vi "Complex to DB.vi"(8 "error in (no error)":errorcluster, 11 "Complix FFT In":refnum<class "2D Array c32.lvclass">) -> (0 "error out":errorcluster, 3 "Db Amplitude Out":refnum<class "2D Array f32.lvclass">)   [LabVIEW 2020, in "Signal Analysis.lvlib" / "Signal Analysis.lvclass"]
uses:
  Signal Analysis.lvclass
  <vilib>/Natan Biesmans/G2CPU GPU and CPU HPC Toolkit/G2CPU Libraries/Arrays/2DArray/c32/2D Array c32.lvclass
  C:/Program Files/National Instruments/LabVIEW 2025/vi.lib/Natan Biesmans/G2CPU GPU and CPU HPC Toolkit/G2CPU Libraries/Arrays/Array/Array Prototype.lvclass
  <vilib>/Natan Biesmans/G2CPU GPU and CPU HPC Toolkit/G2CPU Libraries/Arrays/2DArray/f32/2D Array f32.lvclass
  ae8c32fd-c519-49ae-a133-193997b97273.vi
  5b3a9c71-2296-4b0e-aa5a-23b530eb68bb.vi
  9631c890-40d0-4dd2-8f0c-9650434c6622.vi
  71c5292d-49ae-4f2f-bdc5-1c901a887993.vi
  ae8c32fd-c519-49ae-a133-193997b97273.vi/b6535cc3-4f5d-45ad-9052-c08cd62b0315.vi
  ae8c32fd-c519-49ae-a133-193997b97273.vi/c9d07b13-7729-4cda-a81e-7ca6043257da.vi
  ae8c32fd-c519-49ae-a133-193997b97273.vi/4470c8c9-d353-49e9-bc1e-f4fe0b2204ee.vi
  ae8c32fd-c519-49ae-a133-193997b97273.vi/b48f0110-6046-499d-b6aa-1db73cdea65c.vi
  5b3a9c71-2296-4b0e-aa5a-23b530eb68bb.vi/def40612-844c-421c-bb75-87c330777b0b.vi
  9631c890-40d0-4dd2-8f0c-9650434c6622.vi/31b317ac-79b4-42cb-9c55-b9b94a2bc574.vi
  71c5292d-49ae-4f2f-bdc5-1c901a887993.vi/6197f869-f6d4-49b3-9b2c-cc979b422c2e.vi
  71c5292d-49ae-4f2f-bdc5-1c901a887993.vi/a7e86dbb-b4c0-485c-89c5-522e60ee265c.vi
  71c5292d-49ae-4f2f-bdc5-1c901a887993.vi/6197f869-f6d4-49b3-9b2c-cc979b422c2e.vi/2c12aba4-aacf-4d7a-adbe-039f6155a93e.vi
  71c5292d-49ae-4f2f-bdc5-1c901a887993.vi/6197f869-f6d4-49b3-9b2c-cc979b422c2e.vi/f38cccb2-46f6-49f0-a8d6-9da0c88ff6f3.vi
  71c5292d-49ae-4f2f-bdc5-1c901a887993.vi/6197f869-f6d4-49b3-9b2c-cc979b422c2e.vi/bdde7ba0-fc5a-4512-a8ec-1695e5fcee25.vi
  71c5292d-49ae-4f2f-bdc5-1c901a887993.vi/6197f869-f6d4-49b3-9b2c-cc979b422c2e.vi/3e802c67-fb96-46a3-ae13-4994a8508b4f.vi
  71c5292d-49ae-4f2f-bdc5-1c901a887993.vi/6197f869-f6d4-49b3-9b2c-cc979b422c2e.vi/5a50fc67-79e7-4972-80c2-92243cd53dd4.vi
  71c5292d-49ae-4f2f-bdc5-1c901a887993.vi/a7e86dbb-b4c0-485c-89c5-522e60ee265c.vi/730f6c57-5c0b-4ee9-b61e-75067b25222b.vi
  71c5292d-49ae-4f2f-bdc5-1c901a887993.vi/a7e86dbb-b4c0-485c-89c5-522e60ee265c.vi/096b8799-7810-404e-baca-ba9279cec4bd.vi
  71c5292d-49ae-4f2f-bdc5-1c901a887993.vi/a7e86dbb-b4c0-485c-89c5-522e60ee265c.vi/0f1a5a47-bcc5-4796-ac31-8dfcfbc0d7d1.vi
  71c5292d-49ae-4f2f-bdc5-1c901a887993.vi/a7e86dbb-b4c0-485c-89c5-522e60ee265c.vi/89f12e17-3330-4b72-ad8f-8dd636660732.vi
  71c5292d-49ae-4f2f-bdc5-1c901a887993.vi/6197f869-f6d4-49b3-9b2c-cc979b422c2e.vi/5a50fc67-79e7-4972-80c2-92243cd53dd4.vi/1b7cf390-2ae0-48f3-9bce-03c57eed6ee8.vi
  <vilib>/Natan Biesmans/G2CPU GPU and CPU HPC Toolkit/G2CPU Libraries/Arrays/1DArray/f32/1D Array f32.lvclass
  <vilib>/Natan Biesmans/G2CPU GPU and CPU HPC Toolkit/G2CPU Libraries/Arrays/Array/G2CPU Lock Array.vi
  <vilib>/Natan Biesmans/G2CPU GPU and CPU HPC Toolkit/G2CPU Libraries/Arrays/Array/G2CPU Get Array Pointer.vi
  <vilib>/Natan Biesmans/G2CPU GPU and CPU HPC Toolkit/ArrayFire Driver/VIs/real.vi
  <vilib>/Natan Biesmans/G2CPU GPU and CPU HPC Toolkit/ArrayFire Driver/VIs/imag.vi
  <vilib>/Natan Biesmans/G2CPU GPU and CPU HPC Toolkit/ArrayFire Driver/VIs/hypot.vi
  <vilib>/Natan Biesmans/G2CPU GPU and CPU HPC Toolkit/ArrayFire Driver/VIs/release array.vi
  <vilib>/Natan Biesmans/G2CPU GPU and CPU HPC Toolkit/ArrayFire Driver/VIs/arg.vi
  <vilib>/Natan Biesmans/G2CPU GPU and CPU HPC Toolkit/G2CPU Libraries/Arrays/Array/G2CPU Set Array Pointer.vi
  <vilib>/Natan Biesmans/G2CPU GPU and CPU HPC Toolkit/G2CPU Libraries/Arrays/Array/G2CPU Unlock Array.vi
  <vilib>/Natan Biesmans/G2CPU GPU and CPU HPC Toolkit/ArrayFire Driver/VIs/abs.vi
  <vilib>/Natan Biesmans/G2CPU GPU and CPU HPC Toolkit/ArrayFire Driver/VIs/log10.vi
  <vilib>/Natan Biesmans/G2CPU GPU and CPU HPC Toolkit/ArrayFire Driver/VIs/Run as Multi Device.vi
  <vilib>/Natan Biesmans/G2CPU GPU and CPU HPC Toolkit/G2CPU Libraries/Manage Environment/Find AF DLL.vi
  <vilib>/Natan Biesmans/G2CPU GPU and CPU HPC Toolkit/ArrayFire Driver/subvi/Error Converter (ErrCode or Status).vi
  <vilib>/Natan Biesmans/G2CPU GPU and CPU HPC Toolkit/ArrayFire Driver/VIs/cast.vi
  <vilib>/Natan Biesmans/G2CPU GPU and CPU HPC Toolkit/G2CPU Libraries/Arrays/SubVI/Lock Arrays.vi
  <vilib>/Natan Biesmans/G2CPU GPU and CPU HPC Toolkit/G2CPU Libraries/Arrays/SubVI/is 2D.vi
  <vilib>/Natan Biesmans/G2CPU GPU and CPU HPC Toolkit/ArrayFire Driver/VIs/mul.vi
  <vilib>/Natan Biesmans/G2CPU GPU and CPU HPC Toolkit/G2CPU Libraries/Arrays/Array/Array Prototype.lvclass
  <vilib>/Natan Biesmans/G2CPU GPU and CPU HPC Toolkit/G2CPU Libraries/Arrays/DataTypes/c32/c32.lvclass
  <vilib>/Natan Biesmans/G2CPU GPU and CPU HPC Toolkit/G2CPU Libraries/Arrays/2DArray/2D Array Prototype.lvclass
  <vilib>/Natan Biesmans/G2CPU GPU and CPU HPC Toolkit/G2CPU Libraries/Arrays/DataTypes/f32/f32.lvclass
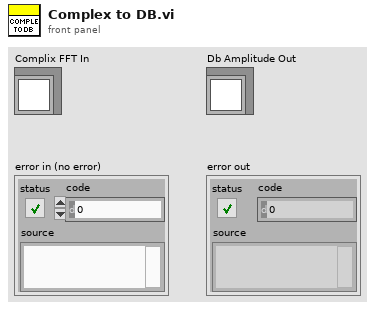
[diagram p1: front panel]
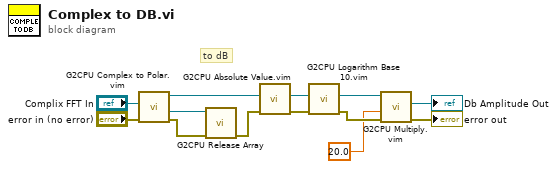
[diagram p0: block diagram]
diagram:
  # "to dB"
  n1 = call "G2CPU Complex to Polar.vim"("error in (no error)"="error in (no error)", "Array Real"="Complix FFT In") -> ("error out"=w1:errorcluster, "Array Theta"=w2:refnum<class "2D Array f32.lvclass">, "Array r"=w3:refnum<class "2D Array f32.lvclass">)  [unwired: 7 in]
  n2 = call <vilib>:"G2CPU Release Array.vi"("error in (no error)"=w1, "Array in"=w2) -> ("error out"=w9:errorcluster)  [unwired: 9 in]
  n3 = call "G2CPU Absolute Value.vim"("error in (no error)"=w9, "Array in"=w3) -> ("error out"=w7:errorcluster, "Array Result"=w8:refnum<class "2D Array f32.lvclass">)  [unwired: 8 in]
  n4 = call "G2CPU Logarithm Base 10.vim"("error in (no error)"=w7, "Array in"=w8) -> ("error out"=w5:errorcluster, "Array Result"=w6:refnum<class "2D Array f32.lvclass">)  [unwired: 8 in]
  n5 = call "G2CPU Multiply.vim"("error in (no error)"=w5, "Array rhs"=sgl 20.0, "Array lhs"=w6) -> ("error out"=→"error out":errorcluster, "Array Result"=→"Db Amplitude Out":refnum<class "2D Array f32.lvclass">)  [unwired: 7 in]
